vi "Practice.vi"() -> ()   [LabVIEW 2021]
panel:
  in  "stop":bool
  in  "Pattern":string(combo)="One white"
  out "Boolean array 3":bool[](array[boolean])
  out "ID":bool
  out "Boolean array 2":bool[](array[boolean])
  out "Boolean array":bool[](array[boolean])
  out "Array":bool[](array[boolean])
  out "Reset":bool
  out "Zero?":bool
  in  "ID 2":u8
  in  "ID":u32
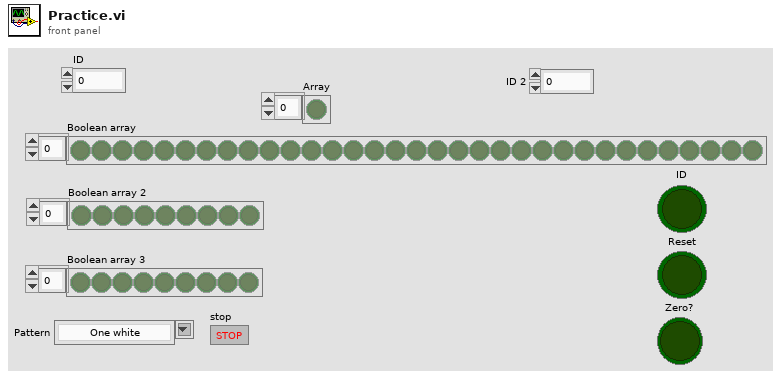
[diagram p1: front panel]
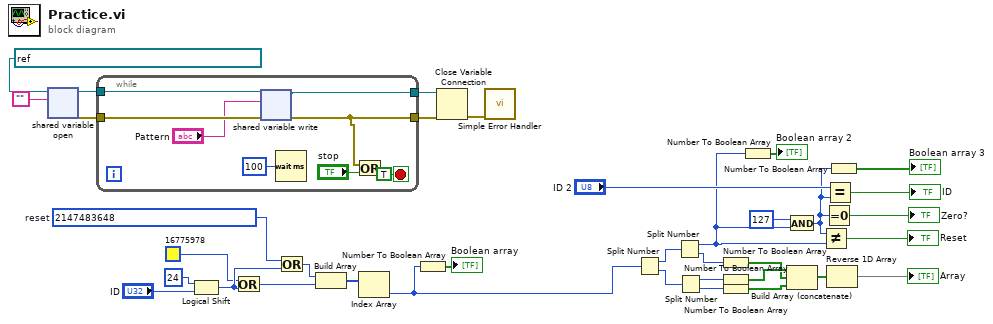
[diagram p0: block diagram]
diagram:
  w18 = u32 2147483648  # reset
  n1 = shared-variable-open(refnum<k21> "ni.var.psp://myrio-1900/Variables/Pattern" ("shared variable refnum in"), "") -> (w7:refnum<k21>, w4:errorcluster)  [unwired: 2 in]
  n2 = while {
    tunnel: w7 -> [w42]
    tunnel: [w41] -> w6
    tunnel: [w39] -> w5
    tunnel: w4 -> [w40]
    stop <- TRUE stop-if-true
    n3 = shared-variable-write(w42, w40, "Pattern") -> (w41:refnum<k21>, w39:errorcluster)
    n4 = Wait (ms)(milliseconds to wait=u32 100) -> ()  [unwired: 1 out]
    n5 = Or(x=w39, y="stop") -> ()  [unwired: 1 out]
  }
  n6 = Logical Shift(y=i16 24, x="ID") -> (x << y=w20:u32)
  n7 = Or(x=u32 16775978, y=w20) -> (x .or. y?=w21:u32)
  n8 = Or(x=w18, y=w20) -> (x .or. y?=w19:u32)
  n9 = Build Array(w19, w21) -> (w17:u32[])
  n10 = Index Array(array=w17) -> (element=w15:u32)  [unwired: 1 in]
  n11 = Number To Boolean Array(number=w15) -> (Boolean array=→"Boolean array":bool[])
  n12 = Close Variable Connection(8:w5, 11:w6) -> (0:w3:errorcluster)
  n13 = call <vilib>:"Simple Error Handler.vi"("error in (no error)"=w3) -> ()  [unwired: 4 in, 5 out]
  n14 = Split Number(x=w15) -> (hi(x)=w31:u16, lo(x)=w30:u16)
  n15 = Split Number(x=w31) -> (hi(x)=w12:u8, lo(x)=w29:u8)
  n16 = Split Number(x=w30) -> (hi(x)=w28:u8, lo(x)=w27:u8)
  n17 = Number To Boolean Array(number=w29) -> (Boolean array=w25:bool[])
  n18 = Number To Boolean Array(number=w28) -> (Boolean array=w26:bool[])
  n19 = Number To Boolean Array(number=w27) -> (Boolean array=w24:bool[])
  n20 = Number To Boolean Array(number=w12) -> (Boolean array=→"Boolean array 2":bool[])
  n21 = And(x=u8 127, y=w12) -> (x .and. y?=w9:u8)
  n22 = Build Array (concatenate)(w26, w25, w24) -> (w23:bool[])
  n23 = Not Equal?(x=w9, y=w12) -> (x != y?=→"Reset":bool)
  n24 = Equal To 0?(x=w9) -> (x = 0?=→"Zero?":bool)
  n25 = Equal?(x="ID 2", y=w9) -> (x = y?=→"ID":bool)
  n26 = Reverse 1D Array(array=w23) -> (reversed array=→"Array":bool[])
  n27 = Number To Boolean Array(number=w9) -> (Boolean array=→"Boolean array 3":bool[])
